vi "例4.1 求两个数的和与差.vi"() -> ()   [LabVIEW 2017]
panel:
  out "y":dbl
  out "x":dbl
  in  "b":dbl
  in  "a":dbl
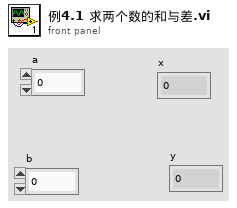
[diagram p1: front panel]
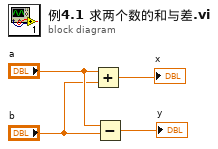
[diagram p0: block diagram]
diagram:
  n1 = Add(x="a", y="b") -> (x+y=→"x":dbl)
  n2 = Subtract(x="a", y="b") -> (x-y=→"y":dbl)
